vi "RunCore.vi"(0 "VI refnum in":refnum<vi>, 5 "Wait until VI done?":bool caption="Wait until VI done? (F)", 7 "Auto dispose VI refnum?":bool=TRUE caption="Auto dispose VI refnum? (T)", 11 "Error in":errorcluster caption="Error in (no error)") -> (4 "VI refnum out":refnum<vi>, 6 "VI running?":bool, 8 "Last execution state":T1(ring), 15 "Error out":errorcluster)   [LabVIEW 2017, in "VILauncher.lvlib"]
doc: "Runs the VI that <B>VI refnum in</B> refers to.\n\nThis function will wait until the VI is done if <B>Wait until VI done?</B> is True (default is False), and it will auto dispose the VI reference (hand it over to the running VI) if <B>Auto dispose VI refnum?</B> is True.\n\nThe VI must already be in memory (execution state \"Idle\" or \"Running\") for this function to take any action.\n\nThe <B>VI running?</B> output will only be True if the VI's <B>Last execution state</B> is \"Run top level\". Note that if this function fails to run the VI, <B>VI refnum in</B> will not be auto-disposed, in which case you retain the responsibility of closing that reference yourself.\n\nThis VI is reentrant, and it doesn't run if there is an error on <B>Error in</B>.\n\nSteen Schmidt\nGPower\n30/12 2012"
uses:
  VILauncher.lvlib
panel:
  # "Copyright © 2013\nSteen Schmidt, GPower\nSee enclosed license file for terms and conditions"
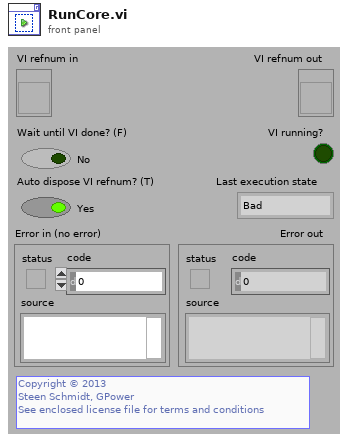
[diagram p1: front panel]
types:
  T1 = enum32{"Bad", "Idle", "Run top level", "Running"}
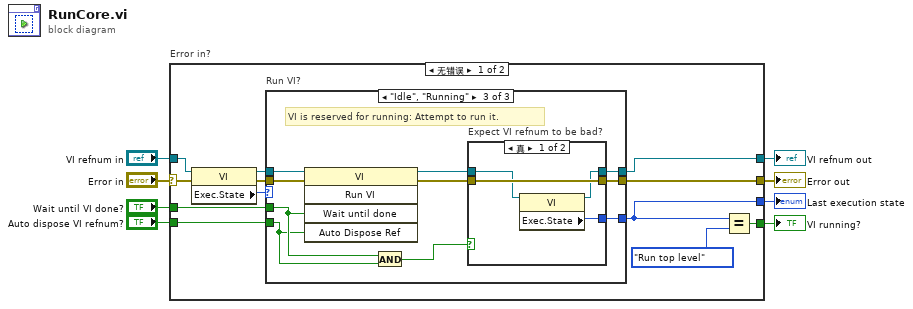
[diagram p0: block diagram]
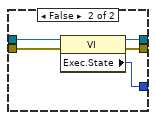
[diagram p4: hidden frame]
diagram:
  n1 = case "Error in?" shown="无错误" "Error in" {
    selector: "Error in" -> [w18 w46]
    tunnel: [w20 w46] -> w7
    tunnel: "VI refnum in" -> [w16 w47]
    tunnel: [w19 w47] -> w5
    tunnel: [w13 _] -> w4
    tunnel: [w11 _] -> w3
    tunnel: "Auto dispose VI refnum?" -> [w10 _]
    tunnel: "Wait until VI done?" -> [w9 _]
    frame No Error {
      n2 = property class="VI"(reference=w16, error in=w18) -> (reference out=w15:refnum<vi>, error out=w17:errorcluster, "Exec.State"=w14:T1)
      n3 = case "Run VI?" shown="\"Idle\", \"Running\"" w14 {
        selector: w14 -> [w21 w24 _]
        tunnel: [w23 w26 w33] -> w20
        tunnel: w17 -> [w23 w26 w36]
        tunnel: w15 -> [w22 w25 w35]
        tunnel: [w22 w25 w31] -> w19
        tunnel: [w21 w24 w30] -> w13
        tunnel: w10 -> [_ _ w28]
        tunnel: w9 -> [_ _ w29]
        frame "Bad" {
          # "VI is not in a state to be started: Do nothing."
        }
        frame "Run top level" {
          # "VI is already running: Do nothing."
        }
        frame "Idle", "Running" {
          # "VI is reserved for running: Attempt to run it."
          n4 = invoke on="Run VI" class="VI" method="Run VI"(reference=w35, error in=w36, "Wait until done"=w29, "Auto Dispose Ref"=w28) -> (reference out=w32:refnum<vi>, error out=w34:errorcluster)  [unwired: 1 in, 3 out]
          n5 = And(x=w29, y=w28) -> (x .and. y?=w27:bool)
          n6 = case "Expect VI refnum to be bad?" shown="真" w27 {
            tunnel: w34 -> [w40 w45]
            tunnel: [w40 w44] -> w33
            tunnel: w32 -> [w39 w43]
            tunnel: [w37 w42] -> w31
            tunnel: [w38 w41] -> w30
            frame True {
              n7 = property class="VI"(reference=w39) -> (reference out=w37:refnum<vi>, "Exec.State"=w38:T1)  [unwired: 1 in, 1 out]
            }
            frame False {
              n8 = property class="VI"(reference=w43, error in=w45) -> (reference out=w42:refnum<vi>, error out=w44:errorcluster, "Exec.State"=w41:T1)
            }
          }
        }
      }
      n9 = Equal?(x=w13, y=T1."Run top level") -> (x = y?=w11:bool)
    }
    frame Error {
    }
  }
  "Error out" <- w7
  "VI refnum out" <- w5
  "Last execution state" <- w4
  "VI running?" <- w3
